vi "eFGV - Restart RT Engine.vi"(6 "Action":T1, 8 "Error In":errorcluster, 11 "Restart RT? In":bool) -> (0 "Error Out":errorcluster, 2 "Event Restart RT":refnum<user-event>, 3 "Restart RT? Out":bool)   [LabVIEW 2020]
uses:
  Control/State - eFGV.ctl
  <vilib>/event_ctls.llb/usereventprio.ctl
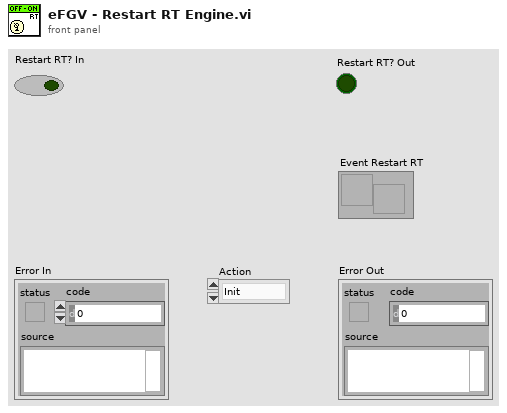
[diagram p1: front panel]
types:
  T1 = typedef "State - eFGV.ctl" = enum16{"Init", "Read", "Write", "Exit"}
  T2 = typedef "usereventprio.ctl" = enum32{"high priority", "normal priority"}
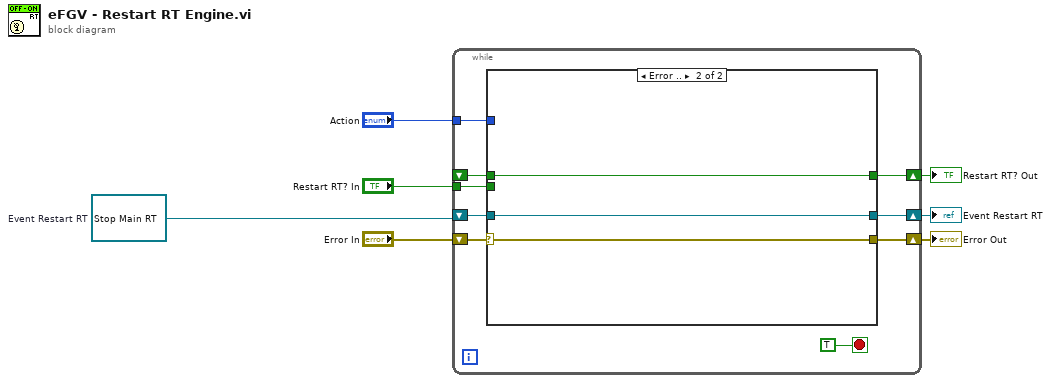
[diagram p0: block diagram]
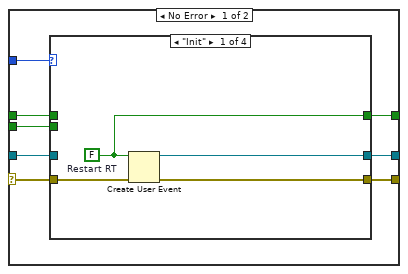
[diagram p2: hidden frame]
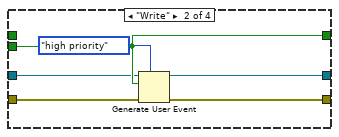
[diagram p3: hidden frame]
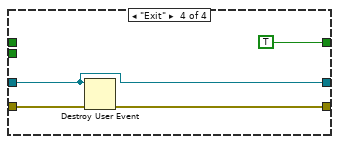
[diagram p5: hidden frame]
diagram:
  w2 = refnum<user-event> refnum  # Event Restart RT
  n1 = while {
    tunnel: "Action" -> [w13]
    shift-right: [w16] -> w7
    shift-left: "Error In" -> [w15]
    tunnel: "Restart RT? In" -> [w12]
    shift-right: [w11] -> w3
    shift-left: _ -> [w10]
    shift-right: [w9] -> w1
    shift-left: w2 -> [w8]
    stop <- TRUE stop-if-true
    n2 = case shown="Error .." w15 {
      selector: w15 -> [w23 w44]
      tunnel: [w24 w44] -> w16
      tunnel: w13 -> [w22 _]
      tunnel: w12 -> [w21 _]
      tunnel: [w20 w43] -> w11
      tunnel: w10 -> [w19 w43]
      tunnel: [w18 w42] -> w9
      tunnel: w8 -> [w17 w42]
      frame No Error {
        n3 = case shown="\"Init\"" w22 {
          tunnel: w23 -> [w28 w34 w37 w41]
          tunnel: [w27 w33 w37 w40] -> w24
          tunnel: w21 -> [_ w32 _ _]
          tunnel: [w26 w32 w36 TRUE ("Stop?")] -> w20
          tunnel: w19 -> [_ _ w36 _]
          tunnel: [w25 w30 w35 w38] -> w18
          tunnel: w17 -> [_ w29 w35 w38]
          frame "Init" {
            w26 = FALSE  # Restart RT
            n4 = Create User Event(user event datatype=w26, error in=w28) -> (user event=w25:refnum<user-event>, error out=w27:errorcluster)
          }
          frame "Write" {
            n5 = Generate User Event(priority (normal)=usereventprio."high priority", user event=w29, event data cluster=w32, error in=w34) -> (user event out=w30:refnum<user-event>, error out=w33:errorcluster)
          }
          frame "Read" {
          }
          frame "Exit" {
            n6 = Destroy User Event(user event=w38, error in=w41) -> (error out=w40:errorcluster)
          }
        }
      }
      frame Error {
      }
    }
  }
  "Error Out" <- w7
  "Restart RT? Out" <- w3
  "Event Restart RT" <- w1
